vi "Application Name--constant.vi"() -> (3 "Application Name":string)   [LabVIEW 2020, in "Application.lvlib"]
doc: "Return the Application name.\n_____\nBased on DQMH Dev Tools: Project Template 7.1.0.1499."
uses:
  Application.lvlib
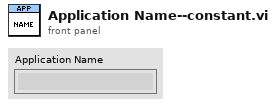
[diagram p1: front panel]
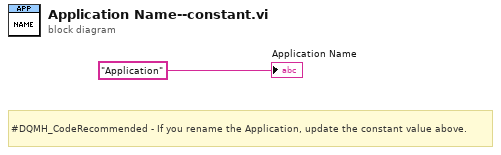
[diagram p0: block diagram]
diagram:
  # "#DQMH_CodeRecommended - If you rename the Application, update the constant value above."
  "Application Name" <- "Application" ("Application Name 2")
